vi "Get All Outgoing Frames.vi"(8 "error in":errorcluster, 11 "Item Ref":T4 format="%.0x") -> (0 "error out":errorcluster, 2 "Frames":T3(array[cluster]) {"Frame Transmit Info"."Transmit Time" format="%#_p"}, 3 "Item Ref out":T4 format="%.0x")   [LabVIEW 2015, in "J1939 Addon System Explorer.lvlib"]
uses:
  J1939 Addon System Explorer.lvlib
  <vilib>/NI Veristand/Custom Device API/Custom Device Item Ref.ctl
  Shared/Types/XNET Frame Event Properties.ctl
  Shared/Types/SPN Properties.ctl
  Shared/SubVIs/Constants.vi
  <vilib>/NI Veristand/Custom Device Tools/Custom Device Utility Library/NI VeriStand - Search for All Items by GUID.vi
  <vilib>/NI Veristand/Custom Device API/Get Item Property (U32).vi
  <vilib>/NI Veristand/Custom Device API/Get Item Property (Variant).vi
  Shared/J1939 Addon Shared.lvlib
  <vilib>/NI Veristand/Custom Device Tools/Custom Device Utility Library/Custom Device Utility Library.lvlib
  <vilib>/NI VeriStand/Custom Device API/Custom Device API.lvlib
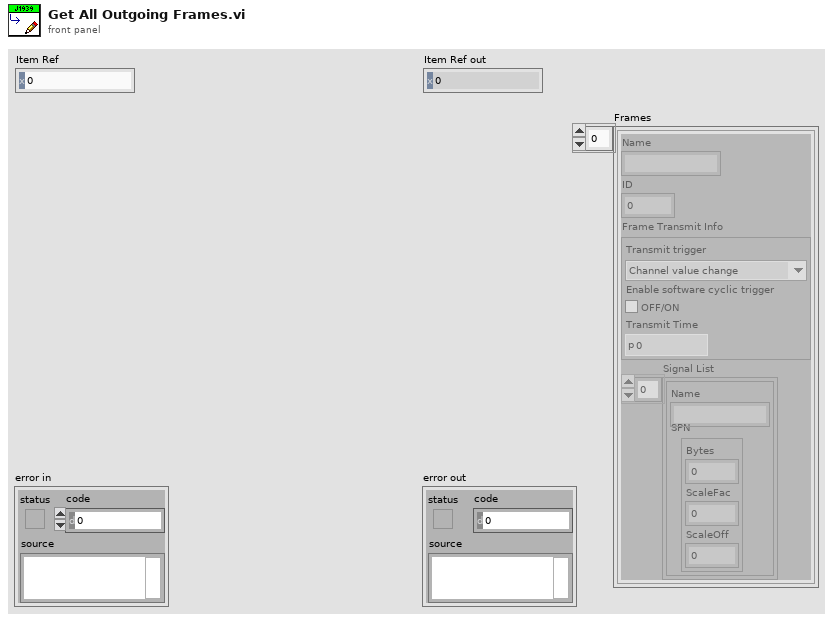
[diagram p1: front panel]
types:
  T1 = typedef "J1939 Addon Shared.lvlib/XNET Frame Event Properties.ctl" = cluster{"Transmit trigger":enum16{"Channel value change"}, "Enable software cyclic trigger":bool, "Transmit Time":dbl}
  T2 = typedef "J1939 Addon Shared.lvlib/SPN Properties.ctl" = cluster{"Bytes":u32, "ScaleFac":dbl, "ScaleOff":dbl}
  T3 = cluster{"Name":string, "ID":u32, "Frame Transmit Info":T1, "Signal List":cluster{"Name":string, "SPN":T2}[]}[]
  T4 = typedef "Custom Device API.lvlib/Custom Device Item Ref.ctl" = u64
  T5 = typedef "Custom Device API.lvlib/Custom Device Item Info.ctl" = cluster{"Name":string, "Is Channel":bool, "GUID":string, "Is Waveform":bool}
  T6 = cluster{"Name":string, "Value":u32, "Cluster":T1, cluster{"Name":string, "cluster":T2}[]}
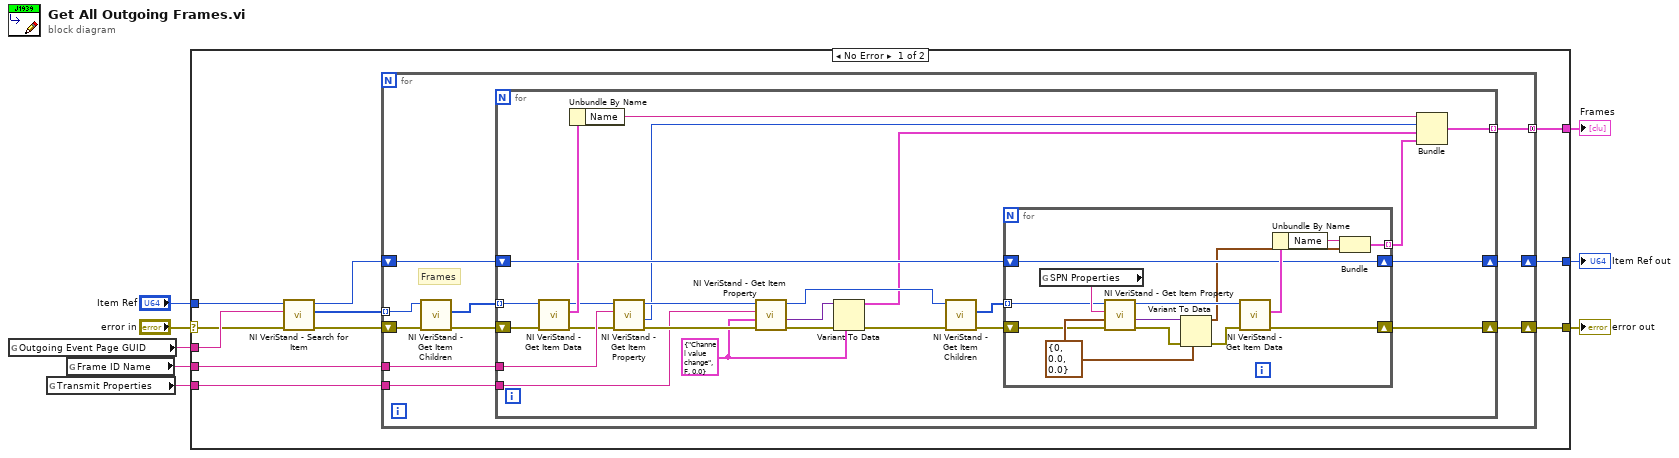
[diagram p0: block diagram]
diagram:
  n1 = global read "Constants.vi" "Outgoing Event Page GUID"() -> (w4:string)
  n2 = global read "Constants.vi" "Transmit Properties"() -> (w2:string)
  n3 = global read "Constants.vi" "Frame ID Name"() -> (w7:string)
  n4 = case shown="No Error" "error in" {
    selector: "error in" -> [w13 w69]
    tunnel: [w10 w68] -> w8
    tunnel: w7 -> [w19 _]
    tunnel: [w11 w69] -> w6
    tunnel: "Item Ref" -> [w12 w68]
    tunnel: w4 -> [w18 _]
    tunnel: w2 -> [w17 _]
    tunnel: [w9 _] -> w1
    frame No Error {
      n5 = call-poly <vilib>:"NI VeriStand - Search for Item.vi"("error in"=w13, "Item GUID"=w18, "Section Ref in"=w12) -> ("error out"=w16:errorcluster, "Item Refs"=w14:T4[], "Section Ref out"=w15:T4)  [unwired: 5 in, 1 out]
      n6 = for {
        tunnel: w19 -> [w29]
        tunnel: w17 -> [w26]
        tunnel: [w24] -> w9 mode=concatenating
        shift-right: [w23] -> w10
        shift-left: w15 -> [w21]
        shift-right: [w25] -> w11
        shift-left: w16 -> [w22]
        tunnel: w14 -> [w20] mode=indexing
        # "Frames"
        n7 = call <vilib>:"NI VeriStand - Get Item Children.vi"("error in (no error)"=w22, "Item Ref in"=w20) -> ("error out"=w27:errorcluster, "Child Refs"=w28:T4[])  [unwired: 6 in, 2 out]
        n8 = for {
          shift-right: [w35] -> w25
          shift-left: w27 -> [w47]
          tunnel: w28 -> [w48] mode=indexing
          tunnel: w29 -> [w53]
          shift-right: [w50] -> w23
          shift-left: w21 -> [w51]
          tunnel: [w32] -> w24 mode=indexing
          tunnel: w26 -> [w41]
          w38 = T1 {"Transmit trigger"=enum."Channel value change", "Enable software cyclic trigger"=FALSE, "Transmit Time"=0.0} ("Cluster")
          n9 = call <vilib>:"NI VeriStand - Get Item Data.vi"("error in (no error)"=w47, "Item Ref in"=w48) -> ("error out"=w44:errorcluster, "Item Info"=w46:T5, "Item Ref out"=w45:T4)  [unwired: 6 in, 1 out]
          n10 = Unbundle By Name(w46) -> ("Name"=w34:string)
          n11 = call-poly <vilib>:"NI VeriStand - Get Item Property.vi"("error in (no error)"=w44, "Property Name"=w53, "Item Ref in"=w45) -> ("error out"=w43:errorcluster, "Value"=w33:u32, "Item Ref out"=w42:T4)  [unwired: 5 in, 1 out]
          n12 = call-poly <vilib>:"NI VeriStand - Get Item Property.vi"("error in (no error)"=w43, "Default Value"=w38, "Property Name"=w41, "Item Ref in"=w42) -> ("error out"=w40:errorcluster, "Value"=w37:variant, "Item Ref out"=w36:T4)  [unwired: 4 in, 1 out]
          n13 = Variant To Data(error in=w40, type=w38, Variant=w37) -> (data=w31:T1, error out=w39:errorcluster)
          n14 = call <vilib>:"NI VeriStand - Get Item Children.vi"("error in (no error)"=w39, "Item Ref in"=w36) -> ("error out"=w52:errorcluster, "Child Refs"=w49:T4[])  [unwired: 6 in, 2 out]
          n15 = for {
            shift-right: [w65] -> w35
            shift-left: w52 -> [w60]
            tunnel: w49 -> [w59] mode=indexing
            shift-right: [w66] -> w50
            shift-left: w51 -> [w66]
            tunnel: [w54] -> w30 mode=indexing
            w61 = T2 {"Bytes"=0, "ScaleFac"=0.0, "ScaleOff"=0.0} ("cluster")
            n16 = global read "Constants.vi" "SPN Properties"() -> (w64:string)
            n17 = call-poly <vilib>:"NI VeriStand - Get Item Property.vi"("error in (no error)"=w60, "Default Value"=w61, "Property Name"=w64, "Item Ref in"=w59) -> ("error out"=w62:errorcluster, "Value"=w63:variant, "Item Ref out"=w58:T4)  [unwired: 4 in, 1 out]
            n18 = Variant To Data(error in=w62, type=w61, Variant=w63) -> (data=w56:T2, error out=w57:errorcluster)
            n19 = call <vilib>:"NI VeriStand - Get Item Data.vi"("error in (no error)"=w57, "Item Ref in"=w58) -> ("error out"=w65:errorcluster, "Item Info"=w67:T5)  [unwired: 6 in, 2 out]
            n20 = Unbundle By Name(w67) -> ("Name"=w55:string)
            n21 = Bundle("Name"=w55, "cluster"=w56) -> (w54:cluster{"Name":string, "cluster":T2})  [unwired: 1 in]
          }
          n22 = Bundle("Name"=w34, "Value"=w33, "Cluster"=w31, w30) -> (w32:T6)  [unwired: 1 in]
        }
      }
    }
    frame Error {
    }
  }
  "error out" <- w6
  "Item Ref out" <- w8
  "Frames" <- w1
